vi "week07_Ex01.vi"() -> ()   [LabVIEW 2017]
panel:
  out "คะแนน":i32
  out "จำนวนรอบที่ทาย":u8
  out "Start":string="เกมเริ่มแล้ว! ทายตัวเลข 1-100"
  out "(มากว่า),(น้อยกว้า),(ถูกต้อง!)":string
  in  "ทายตัวเลขที่สุ่ม":u8
  out "0-100":u8
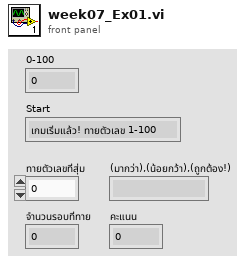
[diagram p1: front panel]
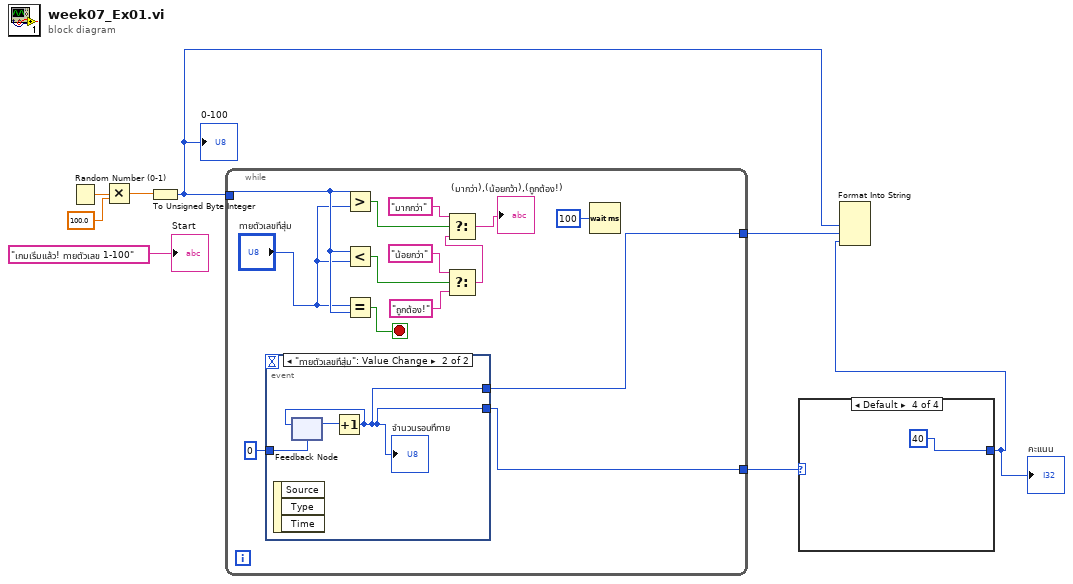
[diagram p0: block diagram]
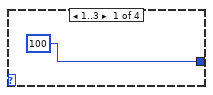
[diagram p2: hidden frame]
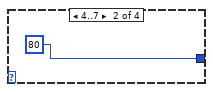
[diagram p3: hidden frame]
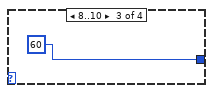
[diagram p4: hidden frame]
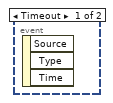
[diagram p5: hidden frame]
diagram:
  n1 = Random Number (0-1)() -> (number: 0 to 1=w8:dbl)
  n2 = Multiply(x=w8, y=100.0) -> (x*y=w6:dbl)
  n3 = To Unsigned Byte Integer(number=w6) -> (unsigned 8bit integer=w5:u8)
  "0-100" <- w5
  n4 = while {
    tunnel: w5 -> [w12]
    tunnel: [w10] -> w3
    tunnel: [w9] -> w2
    stop <- w21 stop-if-true
    n5 = event shown="[1] \"ทายตัวเลขที่สุ่ม\": Value Change" {
      selector: _ -> [_ _]
      dyn-events: _ -> [_ _]
      timeout: _ -> [_ _]
      tunnel: u8 0 ("ทายตัวเลขที่สุ่ม") -> [_ w24]
      tunnel: [_ w23] -> w9
      tunnel: [_ w23] -> w10
      event Timeout {
        n6 = event-data() -> ()  [unwired: 1 in, 3 out]
      }
      event "ทายตัวเลขที่สุ่ม": Value Change {
        n7 = event-data() -> ()  [unwired: 1 in, 3 out]
        n8 = feedback #1(w24) -> (w25:u8)
        n9 = Increment(x=w25) -> (x+1=w23:u8)
        "จำนวนรอบที่ทาย" <- w23
        n10 = feedback-in #1(w23) -> ()
      }
    }
    n11 = Greater?(x=w12, y="ทายตัวเลขที่สุ่ม") -> (0:w19:bool)
    n12 = Less?(x=w12, y="ทายตัวเลขที่สุ่ม") -> (x < y?=w17:bool)
    n13 = Equal?(x="ทายตัวเลขที่สุ่ม", y=w12) -> (x = y?=w21:bool)
    n14 = Select(t="น้อยกว่า", s=w17, f="ถูกต้อง!") -> (s? t:f=w16:string)
    n15 = Select(t="มากกว่า", s=w19, f=w16) -> (s? t:f=→"(มากว่า),(น้อยกว้า),(ถูกต้อง!)":string)
    n16 = Wait (ms)(milliseconds to wait=u32 100) -> ()  [unwired: 1 out]
  }
  n17 = case shown="Default" w2 {
    tunnel: [100 80 60 40] -> w1
    frame 1..3 {
    }
    frame 4..7 {
    }
    frame 8..10 {
    }
    frame Default {
    }
  }
  "คะแนน" <- w1
  n18 = Format Into String(w5, w3, w1) -> ()  [unwired: 3 in, 2 out]
  "Start" <- "เกมเริ่มแล้ว! ทายตัวเลข 1-100"
